vi "Common Path to Specific Path.vi"(4 "common path":string caption="Allgemeiner Pfad") -> (1 "specific path":path caption="Spezifischer Pfad")   [LabVIEW 2009]
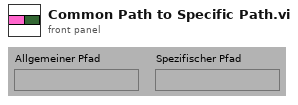
[diagram p1: front panel]
types:
  T1 = enum32{"invalid OS target", "Mac OS", "Windows 3.1", "Windows 95/NT", "Solaris 1", "Solaris 2", "HP-UX", "PowerMAX", "Linux", "Irix", "Rhapsody", "BeOS", "AIX", "OSF1", "VxWorks", "PharLap", "Carbon", "RTX", "Windows x64", "Linux x64"}
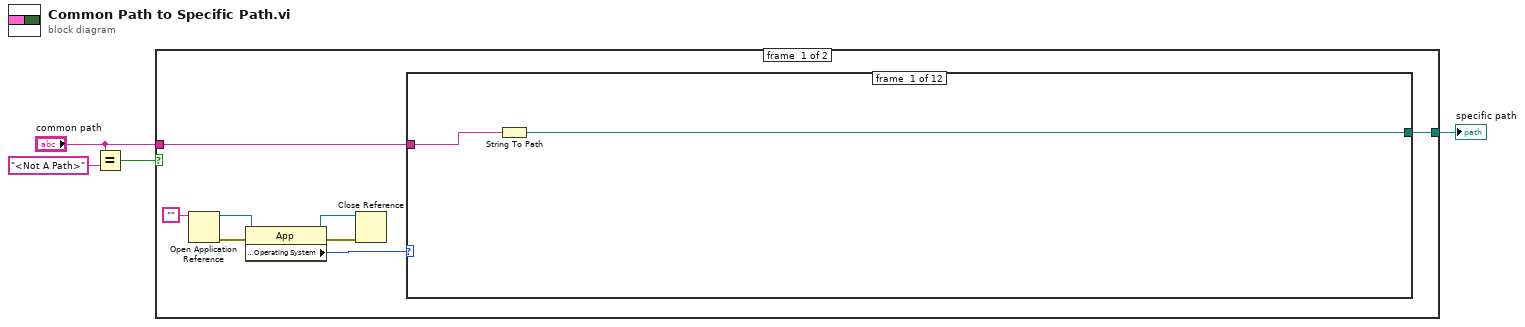
[diagram p0: block diagram]
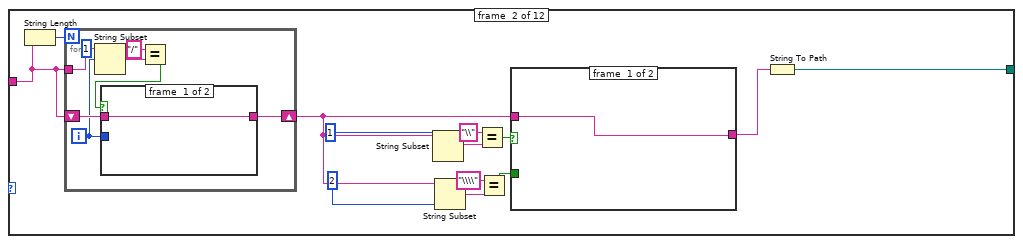
[diagram p2: hidden frame]
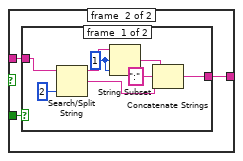
[diagram p3: hidden frame]
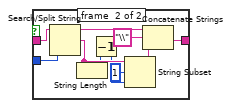
[diagram p5: hidden frame]
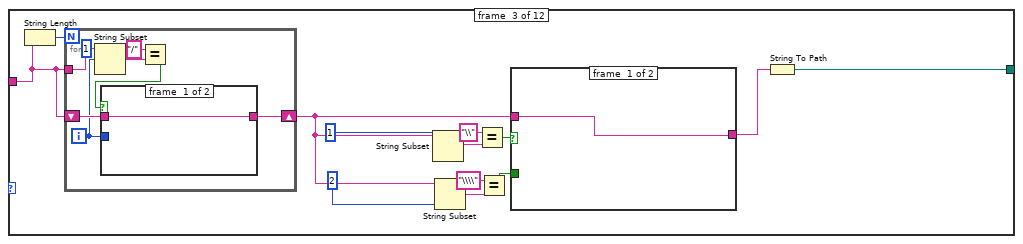
[diagram p6: hidden frame]
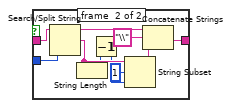
[diagram p7: hidden frame]
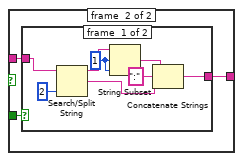
[diagram p8: hidden frame]
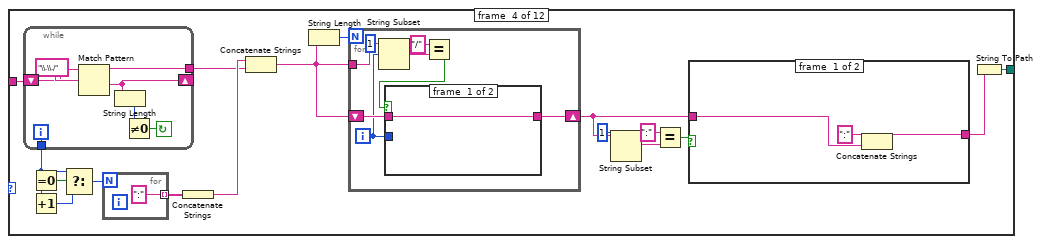
[diagram p10: hidden frame]
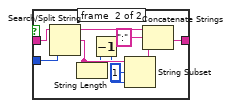
[diagram p11: hidden frame]
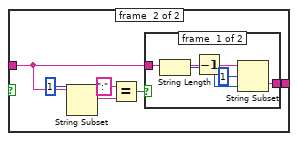
[diagram p12: hidden frame]
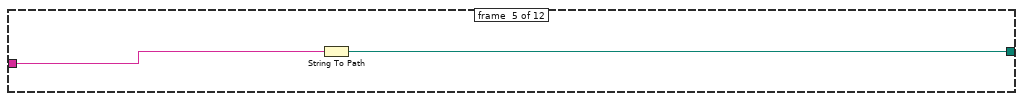
[diagram p14: hidden frame]
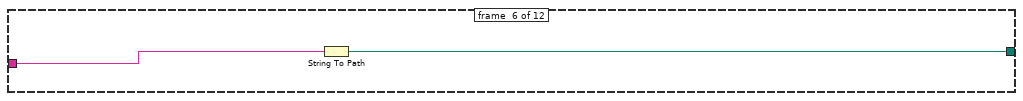
[diagram p15: hidden frame]
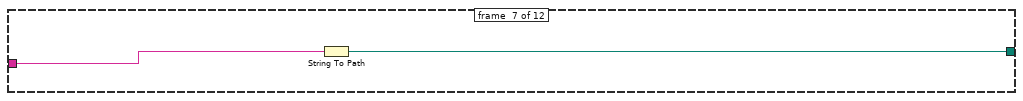
[diagram p16: hidden frame]
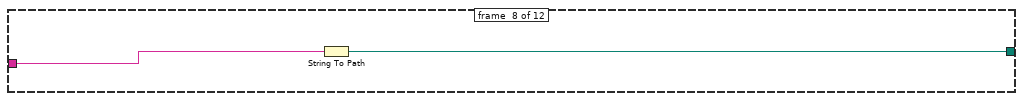
[diagram p17: hidden frame]
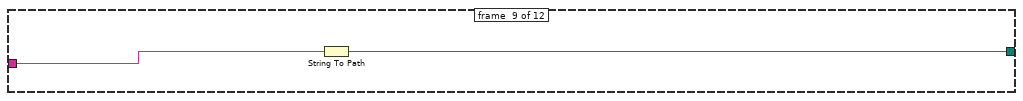
[diagram p18: hidden frame]
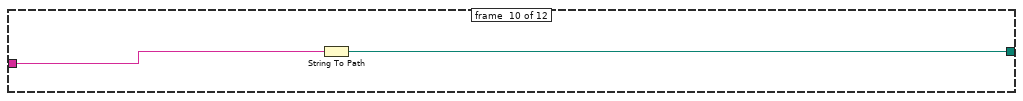
[diagram p19: hidden frame]
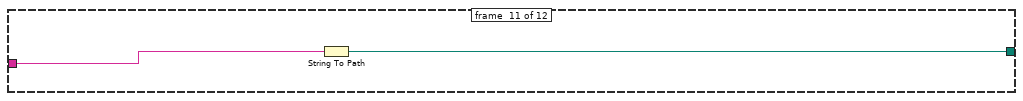
[diagram p20: hidden frame]
diagram:
  n1 = Equal?(x="common path", y="<Not A Path>") -> (x = y?=w1:bool)
  n2 = case shown="False" w1 {
    tunnel: [w12 path ""] -> w4
    tunnel: "common path" -> [w6 _]
    frame #0 {
      n3 = Open Application Reference(11:"") -> (0:w11:errorcluster, 3:w10:refnum<vi>)  [unwired: 3 in]
      n4 = property class="App"(reference=w10, error in=w11) -> (reference out=w8:refnum<vi>, error out=w9:errorcluster, "Application:Target:Operating System"=w5:T1)
      n5 = Close Reference(reference=w8, error in (no error)=w9) -> ()  [unwired: 1 out]
      n6 = case shown="\"Mac OS\", \"Carbon\"" w5 {
        tunnel: w6 -> [w13 w16 w61 w115 w165 w167 w169 w171 w173 w175 w177 w179]
        tunnel: [w14 w27 w72 w121 w164 w166 w168 w170 w172 w174 w176 w178] -> w12
        frame #0 {
          n7 = String To Path(string=w13) -> (path=w14:path)
        }
        frame #1 {
          n8 = String Length(string=w16) -> (length=w17:i32)
          n9 = for {
            N: w17 -> [_]
            tunnel: w16 -> [w46]
            shift-right: [w47] -> w15
            shift-left: w16 -> [w48]
            i -> [w45]
            n10 = String Subset(string=w46, offset (0)=w45, length (rest)=1 ("length")) -> (substring=w43:string)
            n11 = Equal?(x="/", y=w43) -> (x = y?=w41:bool)
            n12 = case shown="True" w41 {
              tunnel: w48 -> [w49 w59]
              tunnel: w45 -> [_ w50]
              tunnel: [w49 w57] -> w47
              frame #0 {
              }
              frame #1 {
                n13 = Search/Split String(string=w59, offset (0)=w50) -> (substring before match=w58:string, match + rest of string=w55:string)  [unwired: 1 in, 1 out]
                n14 = String Length(string=w55) -> (length=w54:i32)
                n15 = Decrement(x=w54) -> (x-1=w53:i32)
                n16 = String Subset(string=w55, offset (0)=1, length (rest)=w53) -> (substring=w51:string)
                n17 = Concatenate Strings(w58, "\\" ("x"), w51) -> (w57:string)
              }
            }
          }
          n18 = String Subset(string=w15, length (rest)=1 ("length")) -> (substring=w25:string)  [unwired: 1 in]
          n19 = String Subset(string=w15, length (rest)=2 ("length")) -> (substring=w20:string)  [unwired: 1 in]
          n20 = Equal?(x="\\", y=w25) -> (x = y?=w23:bool)
          n21 = Equal?(x="\\\\", y=w20) -> (x = y?=w19:bool)
          n22 = case shown="True" w23 {
            tunnel: w15 -> [w28 w31]
            tunnel: [w28 w30] -> w22
            tunnel: w19 -> [_ w29]
            frame #0 {
            }
            frame #1 {
              n23 = case shown="False" w29 {
                tunnel: w31 -> [w39 w40]
                tunnel: [w33 w40] -> w30
                frame #0 {
                  w32 = 1 ("offset (0)")
                  n24 = Search/Split String(string=w39, offset (0)=2) -> (substring before match=w37:string, match + rest of string=w34:string)  [unwired: 1 in, 1 out]
                  n25 = String Subset(string=w37, offset (0)=w32, length (rest)=w32) -> (substring=w36:string)
                  n26 = Concatenate Strings(w36, ":", w34) -> (w33:string)
                }
                frame #1 {
                }
              }
            }
          }
          n27 = String To Path(string=w22) -> (path=w27:path)
        }
        frame #2 {
          n28 = String Length(string=w61) -> (length=w62:i32)
          n29 = for {
            N: w62 -> [_]
            tunnel: w61 -> [w78]
            shift-right: [w79] -> w60
            shift-left: w61 -> [w80]
            i -> [w77]
            n30 = String Subset(string=w78, offset (0)=w77, length (rest)=1 ("length")) -> (substring=w75:string)
            n31 = Equal?(x="/", y=w75) -> (x = y?=w73:bool)
            n32 = case shown="True" w73 {
              tunnel: w80 -> [w81 w91]
              tunnel: w77 -> [_ w82]
              tunnel: [w81 w89] -> w79
              frame #0 {
              }
              frame #1 {
                n33 = Search/Split String(string=w91, offset (0)=w82) -> (substring before match=w90:string, match + rest of string=w87:string)  [unwired: 1 in, 1 out]
                n34 = String Length(string=w87) -> (length=w86:i32)
                n35 = Decrement(x=w86) -> (x-1=w85:i32)
                n36 = String Subset(string=w87, offset (0)=1, length (rest)=w85) -> (substring=w83:string)
                n37 = Concatenate Strings(w90, "\\" ("x"), w83) -> (w89:string)
              }
            }
          }
          n38 = String Subset(string=w60, length (rest)=1 ("length")) -> (substring=w70:string)  [unwired: 1 in]
          n39 = String Subset(string=w60, length (rest)=2 ("length")) -> (substring=w65:string)  [unwired: 1 in]
          n40 = Equal?(x="\\", y=w70) -> (x = y?=w68:bool)
          n41 = Equal?(x="\\\\", y=w65) -> (x = y?=w64:bool)
          n42 = case shown="True" w68 {
            tunnel: w60 -> [w92 w95]
            tunnel: [w92 w94] -> w67
            tunnel: w64 -> [_ w93]
            frame #0 {
            }
            frame #1 {
              n43 = case shown="False" w93 {
                tunnel: w95 -> [w103 w104]
                tunnel: [w97 w104] -> w94
                frame #0 {
                  w96 = 1 ("offset (0)")
                  n44 = Search/Split String(string=w103, offset (0)=2) -> (substring before match=w101:string, match + rest of string=w98:string)  [unwired: 1 in, 1 out]
                  n45 = String Subset(string=w101, offset (0)=w96, length (rest)=w96) -> (substring=w100:string)
                  n46 = Concatenate Strings(w100, ":", w98) -> (w97:string)
                }
                frame #1 {
                }
              }
            }
          }
          n47 = String To Path(string=w67) -> (path=w72:path)
        }
        frame #3 {
          n48 = while {
            tunnel: [w122] -> w113
            tunnel: [w124] -> w108
            shift-left: w115 -> [w127]
            shift-right: [w123] -> _
            i -> [w122]
            stop <- w125 continue-if-true
            n49 = Match Pattern(string=w127, regular expression="\\.\\./") -> (before substring=w124:string, after substring=w123:string)  [unwired: 1 in, 2 out]
            n50 = String Length(string=w123) -> (length=w126:i32)
            n51 = Not Equal To 0?(x=w126) -> (x != 0?=w125:bool)
          }
          n52 = Equal To 0?(x=w113) -> (x = 0?=w114:bool)
          n53 = Increment(x=w113) -> (x+1=w112:i32)
          n54 = Select(t=w113, s=w114, f=w112) -> (s? t:f=w111:i32)
          n55 = for {
            N: w111 -> [_]
            tunnel: [":"] -> w110 mode=indexing
          }
          n56 = Concatenate Strings(w110) -> (w109:string)
          n57 = Concatenate Strings(w109, w108) -> (w105:string)
          n58 = String Length(string=w105) -> (length=w107:i32)
          n59 = for {
            N: w107 -> [_]
            tunnel: w105 -> [w134]
            shift-right: [w135] -> w106
            shift-left: w105 -> [w136]
            i -> [w133]
            n60 = String Subset(string=w134, offset (0)=w133, length (rest)=1 ("length")) -> (substring=w131:string)
            n61 = Equal?(x="/", y=w131) -> (x = y?=w129:bool)
            n62 = case shown="True" w129 {
              tunnel: w136 -> [w137 w147]
              tunnel: w133 -> [_ w138]
              tunnel: [w137 w145] -> w135
              frame #0 {
              }
              frame #1 {
                n63 = Search/Split String(string=w147, offset (0)=w138) -> (substring before match=w146:string, match + rest of string=w143:string)  [unwired: 1 in, 1 out]
                n64 = String Length(string=w143) -> (length=w142:i32)
                n65 = Decrement(x=w142) -> (x-1=w141:i32)
                n66 = String Subset(string=w143, offset (0)=1, length (rest)=w141) -> (substring=w139:string)
                n67 = Concatenate Strings(w146, ":" ("x"), w139) -> (w145:string)
              }
            }
          }
          n68 = String Subset(string=w106, length (rest)=1 ("length")) -> (substring=w120:string)  [unwired: 1 in]
          n69 = Equal?(x=":", y=w120) -> (x = y?=w118:bool)
          n70 = case shown="True" w118 {
            tunnel: w106 -> [w151 w154]
            tunnel: [w150 w157] -> w116
            frame #0 {
              n71 = Concatenate Strings(":", w151) -> (w150:string)
            }
            frame #1 {
              w152 = 1 ("length")
              n72 = String Subset(string=w154, offset (0)=w152, length (rest)=w152) -> (substring=w155:string)
              n73 = Equal?(x=":", y=w155) -> (x = y?=w153:bool)
              n74 = case shown="True" w153 {
                tunnel: w154 -> [w159 w163]
                tunnel: [w158 w163] -> w157
                frame #0 {
                  n75 = String Length(string=w159) -> (length=w161:i32)
                  n76 = Decrement(x=w161) -> (x-1=w160:i32)
                  n77 = String Subset(string=w159, offset (0)=1, length (rest)=w160) -> (substring=w158:string)
                }
                frame #1 {
                }
              }
            }
          }
          n78 = String To Path(string=w116) -> (path=w121:path)
        }
        frame #4 {
          n79 = String To Path(string=w165) -> (path=w164:path)
        }
        frame #5 {
          n80 = String To Path(string=w167) -> (path=w166:path)
        }
        frame #6 {
          n81 = String To Path(string=w169) -> (path=w168:path)
        }
        frame #7 {
          n82 = String To Path(string=w171) -> (path=w170:path)
        }
        frame #8 {
          n83 = String To Path(string=w173) -> (path=w172:path)
        }
        frame #9 {
          n84 = String To Path(string=w175) -> (path=w174:path)
        }
        frame #10 {
          n85 = String To Path(string=w177) -> (path=w176:path)
        }
        frame #11 {
          n86 = String To Path(string=w179) -> (path=w178:path)
        }
      }
    }
    frame #1 {
    }
  }
  "specific path" <- w4
